vi "MeasureSerialize.vi"(8 "error in":errorcluster, 9 "OwningElement in":refnum<k20>, 10 "Document in":refnum<k20>, 11 "Measure in":refnum<class "Measure.lvclass">) -> (0 "error out":errorcluster, 1 "OwningElement out":refnum<k20>, 2 "Document out":refnum<k20>, 3 "Measure out":refnum<class "Measure.lvclass">, 4 "Element":refnum<k20>)   [LabVIEW 2021, in "ProligentXMLGenerator.lvlib" / "Measure.lvclass"]
uses:
  Measure.lvclass
  Measure.lvclass/Measure.ctl
  Base/DOMSupport/DOMSupport.lvlib
  Base/Guid/Guid.lvclass
  C:/Projects/proligent-xml-generator-labview/src/ProligentXMLGenerator/Base/NonEmptyString/NonEmptyString.lvclass
  C:/Projects/proligent-xml-generator-labview/src/ProligentXMLGenerator/Base/String/String.lvclass
  C:/Projects/proligent-xml-generator-labview/src/ProligentXMLGenerator/Base/Attribute/Attribute.lvclass
  C:/Projects/proligent-xml-generator-labview/src/ProligentXMLGenerator/Base/Guid/Guid.lvclass
  Base/DateTime/DateTime.lvclass
  C:/Projects/proligent-xml-generator-labview/src/ProligentXMLGenerator/Base/DateTime/DateTime.lvclass
  Base/NonNullableString_TruncateAt_255/NonNullableString_TruncateAt_255.lvclass
  C:/Projects/proligent-xml-generator-labview/src/ProligentXMLGenerator/Base/NonNullableString/NonNullableString.lvclass
  C:/Projects/proligent-xml-generator-labview/src/ProligentXMLGenerator/Base/NonNullableString_TruncateAt_255/NonNullableString_TruncateAt_255.lvclass
  Base/NonEmptyString_30/NonEmptyString_30.lvclass
  C:/Projects/proligent-xml-generator-labview/src/ProligentXMLGenerator/Base/NonEmptyString_30/NonEmptyString_30.lvclass
  Base/NonEmptyString_20/NonEmptyString_20.lvclass
  C:/Projects/proligent-xml-generator-labview/src/ProligentXMLGenerator/Base/NonEmptyString_20/NonEmptyString_20.lvclass
  Base/ExecutionStatus/ExecutionStatus.lvclass
  C:/Projects/proligent-xml-generator-labview/src/ProligentXMLGenerator/Base/ExecutionStatus/ExecutionStatus.lvclass
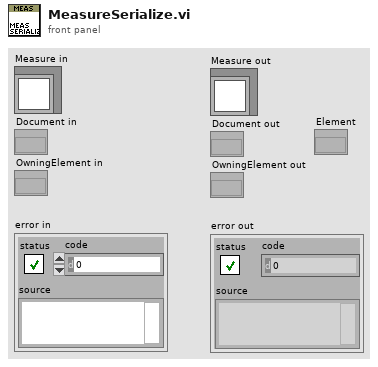
[diagram p1: front panel]
types:
  T1 = typedef "ProligentXMLGenerator.lvlib/Measure.lvclass/Data.ctl" = cluster{"Name":string, "Type":refnum<class "MeasureKind.lvclass">, "Precision":refnum<class "UnsignedByte.lvclass">, "Limit":refnum<class "MeasureLimit.lvclass">, "Characteristics":refnum<class "Characteristic.lvclass">[], "FailureReferences":refnum<class "FailureReference.lvclass">[], "CustomData":refnum<class "CustomData.lvclass">, "MeasureId":refnum<class "Guid.lvclass">, "MeasureTime":refnum<class "DateTime.lvclass">, "Comments":refnum<class "NonNullableString_TruncateAt_255.lvclass">, "Unit":refnum<class "NonEmptyString_30.lvclass">, "Symbol":refnum<class "NonEmptyString_20.lvclass">, "MeasureExecutionStatus":refnum<class "ExecutionStatus.lvclass">}
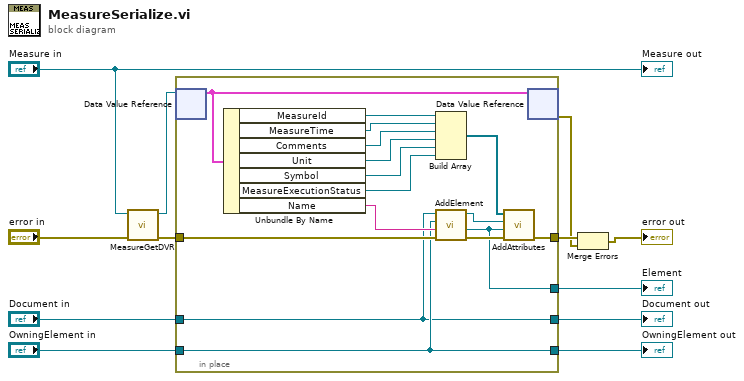
[diagram p0: block diagram]
diagram:
  n1 = call "MeasureGetDVR.vi"("error in"="error in", "Measure"="Measure in") -> ("error out"=w4:errorcluster, "DVRReference"=w3:refnum<data-value>)  [unwired: 8 in]
  n2 = in-place "In Place Element Structure" {
    in-place-border: [w15] -> w5
    in-place-border: "Document in" -> [w24]
    in-place-border: w4 -> [w28]
    in-place-border: "OwningElement in" -> [w26]
    in-place-border: [w26] -> w7
    in-place-border: [w24] -> w6
    in-place-border: [w13] -> w1
    n3 = in-place-dvr #1(w3) -> (w25:T1)  [unwired: 1 out]
    n4 = Unbundle By Name(w25) -> ("MeasureId"=w17:refnum<class "Guid.lvclass">, "MeasureTime"=w19:refnum<class "DateTime.lvclass">, "Comments"=w16:refnum<class "NonNullableString_TruncateAt_255.lvclass">, "Unit"=w18:refnum<class "NonEmptyString_30.lvclass">, "Symbol"=w23:refnum<class "NonEmptyString_20.lvclass">, "MeasureExecutionStatus"=w22:refnum<class "ExecutionStatus.lvclass">, "Name"=w27:string)
    n5 = Build Array(w17, w19, w16, w18, w23, w22) -> (w20:refnum<class "Attribute.lvclass">[])
    n6 = call "AddElement.vi"("error in"=w28, "Name"=w27, "OwningElement in"=w26, "Document in"=w24) -> ("error out"=w21:errorcluster, "NewElement"=w13:refnum<k20>, "Document out"=w14:refnum<k20>)  [unwired: 4 in, 1 out]
    n7 = call "AddAttributes.vi"("error in"=w21, "OwningElement in"=w13, "Document in"=w14, "Attributes"=w20) -> ("error out"=w15:errorcluster)  [unwired: 5 in, 2 out]
    n8 = in-place-dvr #1(w25) -> (w2:errorcluster)  [unwired: 1 out]
  }
  "Document out" <- w6
  "OwningElement out" <- w7
  "Element" <- w1
  n9 = Merge Errors(w5, w2) -> (→"error out":errorcluster)
  "Measure out" <- "Measure in"
